vi "Create Panel by Type.vi"(7 "Panel Type":refnum<class "Panel.lvclass">, 8 "error in (no error)":errorcluster, 9 "Run? (T)":bool=TRUE, 11 "Manager in":refnum<class "Manager.lvclass">) -> (0 "error out":errorcluster, 2 "Panel":refnum<class "Panel.lvclass">, 3 "Manager out":refnum<class "Manager.lvclass">)   [LabVIEW 2020, in "OOPanel.lvlib" / "Manager.lvclass"]
uses:
  Manager.lvclass
  Panel/Panel.lvclass
  Manager.lvclass/Manager.ctl
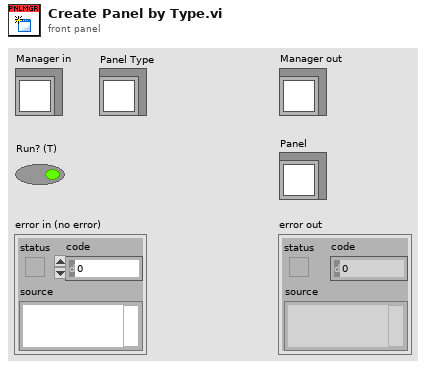
[diagram p1: front panel]
types:
  T1 = typedef "OOPanel.lvlib/Manager.lvclass/Ref Data.ctl" = cluster{"Created Panels":refnum<class "Panel.lvclass">[], "Subpanel Map":map{refnum<vi>, T2}}
  T2 = typedef "OOPanel.lvlib/Manager.lvclass/Subpanel Data.ctl" = cluster{"Panel":refnum<class "Panel.lvclass">, "Has Panel":bool, "Visible":bool}
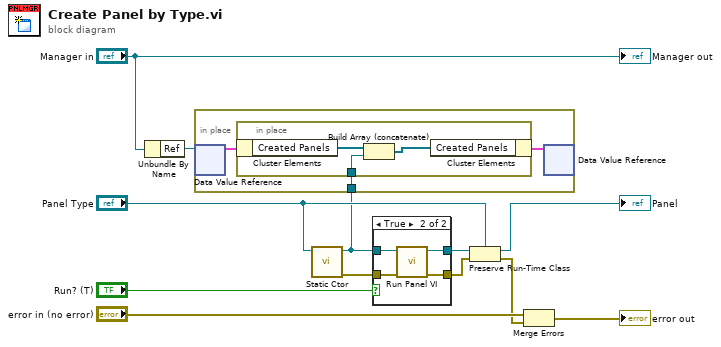
[diagram p0: block diagram]
diagram:
  n1 = Unbundle By Name("Manager in") -> ("Ref"=w5:refnum<data-value>)
  n2 = call "Static Ctor.vi"("Panel in"="Panel Type") -> ("error out"=w4:errorcluster, "Panel out"=w3:refnum<class "Panel.lvclass">)  [unwired: 9 in]
  n3 = in-place {
    in-place-border: w3 -> [w13]
    n4 = in-place-dvr #1(w5) -> (w15:T1)  [unwired: 1 out]
    n5 = in-place {
      in-place-border: w13 -> [w17]
      n6 = in-place-cluster #2(w15) -> ("Created Panels"=w18:refnum<class "Panel.lvclass">[])
      n7 = Build Array (concatenate)(w18, w17) -> (w16:refnum<class "Panel.lvclass">[])
      n8 = in-place-cluster #2("Created Panels"=w16) -> (w14:T1)
    }
    n9 = in-place-dvr #1(w14) -> ()  [unwired: 2 out]
  }
  n10 = case shown="True" "Run? (T)" {
    tunnel: w4 -> [w19 w24]
    tunnel: w3 -> [w20 w23]
    tunnel: [w20 w22] -> w2
    tunnel: [w19 w21] -> w1
    frame False {
    }
    frame True {
      n11 = call "Run Panel VI.vi"("error in (no error)"=w24, "Panel in"=w23) -> ("error out"=w21:errorcluster, "Panel out"=w22:refnum<class "Panel.lvclass">)  [unwired: 8 in]
    }
  }
  n12 = Preserve Run-Time Class(object in=w2, error in=w1, 2:"Panel Type") -> (object out=→"Panel":refnum<class "Panel.lvclass">, error out=w8:errorcluster)
  n13 = Merge Errors("error in (no error)", w8) -> (→"error out":errorcluster)
  "Manager out" <- "Manager in"
